vi "Update Signal Result.vi"(0 "reference in":refnum<class "Reporter.lvclass">, 1 "signal":T1, 2 "pass?":bool, 5 "error in (no error)":errorcluster) -> (14 "reference out":refnum<class "Reporter.lvclass">, 19 "error out":errorcluster)   [LabVIEW 2020, in "Reporter.lvclass"]
uses:
  Reporter.lvclass
  controls/IO Signal List.ctl
  Signal Result.ctl
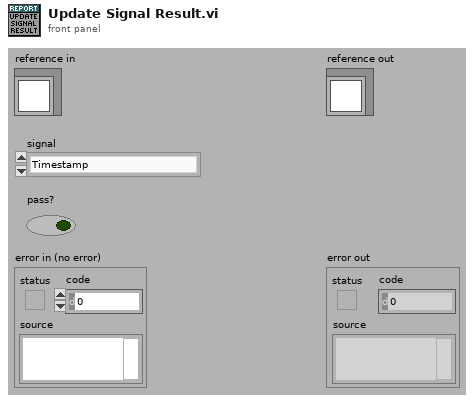
[diagram p1: front panel]
types:
  T1 = typedef "IO Signal List.ctl" = enum16{"Timestamp", "PSU_FB_U_VDC", "PSU_FB_I_AMP", "PSU_FB_W_WATT", "PSU_CMD_U_VDC", "PSU_CMD_I_AMP", "PSU_CMD_OUTPUT", "LCR_PRIMARY", "LCR_SECONDARY", "UV_R_Ohm", "UW_R_Ohm", "VW_R_Ohm", "UV_L_H", "UW_L_H", "VW_L_H", "U_U_VDC", "V_U_VDC", "W_U_VDC", "U_I_AMP", "V_I_AMP", "W_I_AMP", "PWM_CMD_DC_%", "PWM_CMD_VDC", "PWM_CMD_Hz", "PWM_FB_DC_%", "PWM_FB_VDC", "PWM_FB_Hz", "DO_RELAY_U_LCR_A", "DO_RELAY_V_LCR_A", "DO_RELAY_V_LCR_B", "DO_RELAY_W_LCR_B", "DIFF_UV_UW_L_H", "DIFF_UV_VW_L_H", "DIFF_UW_VW_L_H", "DIFF_UV_UW_R_Ohm", "DIFF_UV_VW_R_Ohm", "DIFF_UW_VW_R_Ohm", "DIFF_UV_U_VDC", "DIFF_UW_U_VDC", "DIFF_VW_U_VDC"}
  T2 = typedef "Reporter.lvclass/Signal Result.ctl" = cluster{"signal":T1, "pass?":bool}
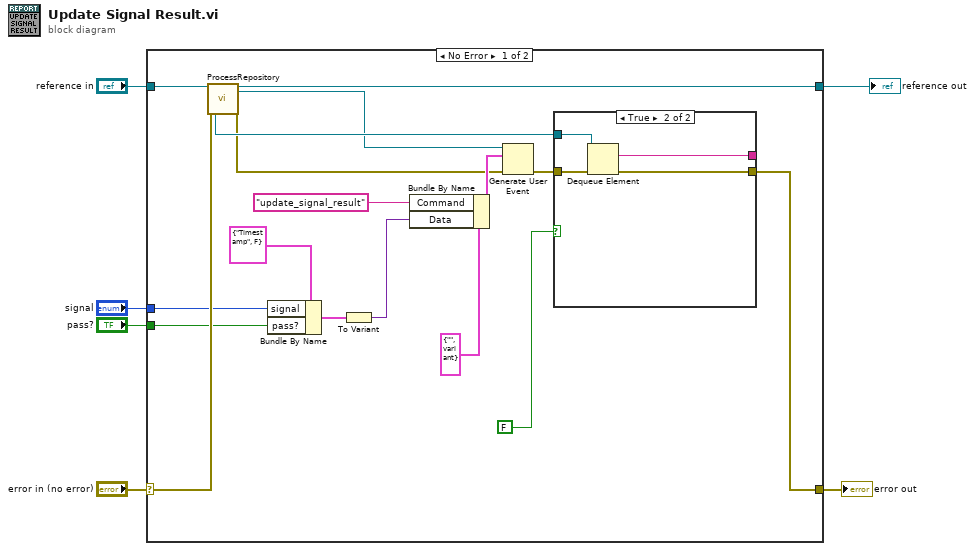
[diagram p0: block diagram]
diagram:
  n1 = case shown="No Error" "error in (no error)" {
    selector: "error in (no error)" -> [w15 w30]
    tunnel: [w13 w30] -> w5
    tunnel: [w14 w29] -> w3
    tunnel: "reference in" -> [w16 w29]
    tunnel: "signal" -> [w11 _]
    tunnel: "pass?" -> [w10 _]
    frame No Error {
      n2 = call "ProcessRepository.vi"("reference in"=w16, "error in (no error)"=w15) -> ("QueueFromProcess"=w23:refnum<queue>, "reference out"=w14:refnum<class "Reporter.lvclass">, "EventsToProcess"=w19:refnum<user-event>, "error out"=w21:errorcluster)  [unwired: 10 in, 4 out]
      n3 = Bundle By Name(cluster=T2 {"signal"=enum."Timestamp", "pass?"=FALSE}, "signal"=w11, "pass?"=w10) -> (w9:T2)
      n4 = To Variant(anything=w9) -> (Variant=w8:variant)
      n5 = Bundle By Name(cluster=cluster{"Command":string, "Data":variant} {"Command"="", "Data"=variant} ("MessageToProcess"), "Command"="update_signal_result", "Data"=w8) -> (w22:cluster{"Command":string, "Data":variant})
      n6 = Generate User Event(user event=w19, event data cluster=w22, error in=w21) -> (error out=w20:errorcluster)  [unwired: 1 in, 1 out]
      n7 = case shown="True" FALSE {
        tunnel: w20 -> [w24 w28]
        tunnel: [_ w27] -> _
        tunnel: [w24 w26] -> w13
        tunnel: w23 -> [_ w25]
        frame False {
        }
        frame True {
          n8 = Dequeue Element(queue=w25, error in (no error)=w28) -> (element=w27:string, error out=w26:errorcluster)  [unwired: 1 in, 2 out]
        }
      }
    }
    frame Error {
    }
  }
  "error out" <- w5
  "reference out" <- w3
